vi "基础16.vi"() -> ()   [LabVIEW 2014]
panel:
  out "数组":dbl[][](array[numeric])
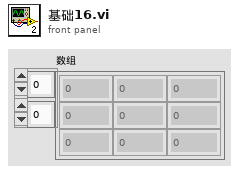
[diagram p1: front panel]
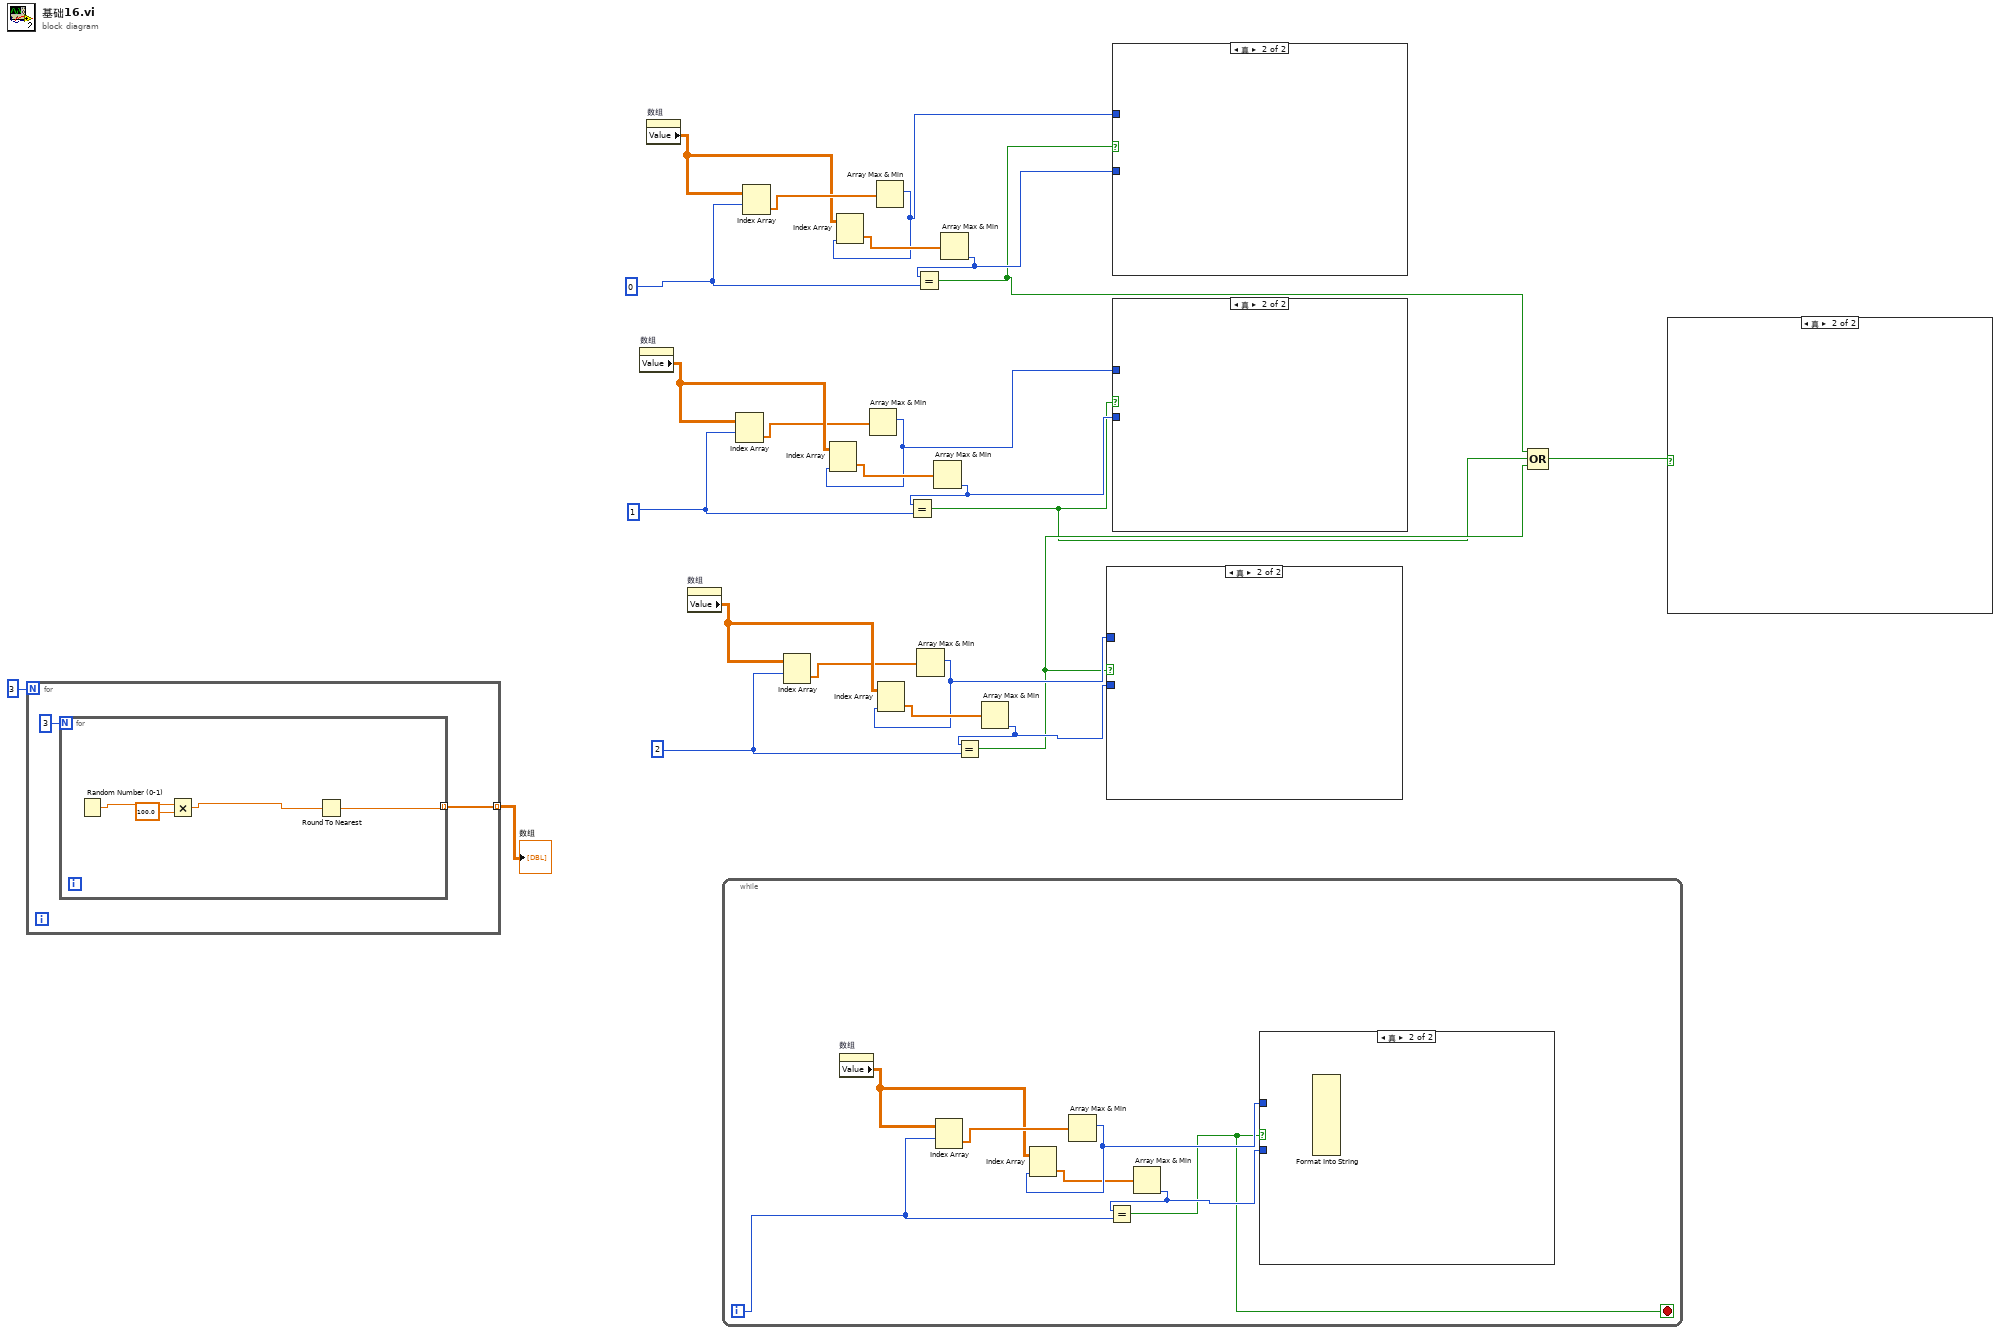
[diagram p0: block diagram]
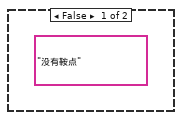
[diagram p3: hidden frame]
diagram:
  w11 = 2
  w12 = 1
  w13 = 0
  n1 = for {
    N: 3 -> [_]
    tunnel: [w25] -> w23 mode=indexing
    n2 = for {
      N: 3 -> [_]
      tunnel: [w27] -> w25 mode=indexing
      n3 = Random Number (0-1)() -> (number: 0 to 1=w30:dbl)
      n4 = Multiply(x=w30, y=100.0) -> (x*y=w28:dbl)
      n5 = Round To Nearest(number=w28) -> (nearest integer value=w27:dbl)
    }
  }
  "数组" <- w23
  n6 = property on="数组" class="Arr (严格)"() -> ("Value"=w15:dbl[][])  [unwired: 2 in, 2 out]
  n7 = property on="数组" class="Arr (严格)"() -> ("Value"=w18:dbl[][])  [unwired: 2 in, 2 out]
  n8 = property on="数组" class="Arr (严格)"() -> ("Value"=w21:dbl[][])  [unwired: 2 in, 2 out]
  n9 = while {
    i -> [w32]
    stop <- w31 stop-if-true
    n10 = property on="数组" class="Arr (严格)"() -> ("Value"=w34:dbl[][])  [unwired: 2 in, 2 out]
    n11 = Index Array(array=w34, index (row)=w32) -> (element=w35:dbl[])  [unwired: 1 in]
    n12 = Array Max & Min(array=w35) -> (max index (indices)=w36:i32)  [unwired: 3 out]
    n13 = Index Array(array=w34, index (col)=w36) -> (element=w33:dbl[])  [unwired: 1 in]
    n14 = Array Max & Min(array=w33) -> (min index (indices)=w37:i32)  [unwired: 3 out]
    n15 = Equal?(x=w37, y=w32) -> (x = y?=w31:bool)
    n16 = case shown="真" w31 {
      tunnel: w36 -> [_ _]
      tunnel: w37 -> [_ _]
      frame False {
      }
      frame True {
        n17 = Format Into String() -> (resulting string=w38:string)  [unwired: 12 in, 1 out]
      }
    }
  }
  n18 = Index Array(array=w15, index (row)=w12) -> (element=w14:dbl[])  [unwired: 1 in]
  n19 = Index Array(array=w18, index (row)=w13) -> (element=w19:dbl[])  [unwired: 1 in]
  n20 = Index Array(array=w21, index (row)=w11) -> (element=w20:dbl[])  [unwired: 1 in]
  n21 = Array Max & Min(array=w14) -> (max index (indices)=w7:i32)  [unwired: 3 out]
  n22 = Index Array(array=w15, index (col)=w7) -> (element=w16:dbl[])  [unwired: 1 in]
  n23 = Array Max & Min(array=w19) -> (max index (indices)=w5:i32)  [unwired: 3 out]
  n24 = Index Array(array=w18, index (col)=w5) -> (element=w17:dbl[])  [unwired: 1 in]
  n25 = Array Max & Min(array=w20) -> (max index (indices)=w10:i32)  [unwired: 3 out]
  n26 = Index Array(array=w21, index (col)=w10) -> (element=w22:dbl[])  [unwired: 1 in]
  n27 = Array Max & Min(array=w16) -> (min index (indices)=w8:i32)  [unwired: 3 out]
  n28 = Equal?(x=w8, y=w12) -> (x = y?=w2:bool)
  n29 = Array Max & Min(array=w17) -> (min index (indices)=w6:i32)  [unwired: 3 out]
  n30 = Equal?(x=w6, y=w13) -> (x = y?=w1:bool)
  n31 = Array Max & Min(array=w22) -> (min index (indices)=w9:i32)  [unwired: 3 out]
  n32 = Equal?(x=w9, y=w11) -> (x = y?=w3:bool)
  n33 = case shown="真" w3 {
    tunnel: w10 -> [_ _]
    tunnel: w9 -> [_ _]
    frame False {
    }
    frame True {
    }
  }
  n34 = case shown="真" w1 {
    tunnel: w5 -> [_ _]
    tunnel: w6 -> [_ _]
    frame False {
    }
    frame True {
    }
  }
  n35 = case shown="真" w2 {
    tunnel: w7 -> [_ _]
    tunnel: w8 -> [_ _]
    frame False {
    }
    frame True {
    }
  }
  n36 = Compound Arithmetic op=OR(w1, w2, w3) -> (w4:bool)
  n37 = case shown="真" w4 {
    frame False {
      w39 = "没有鞍点"
    }
    frame True {
    }
  }
